vi "monitor_center.vi"() -> (1 "yc":dbl, 2 "xc":dbl)   [LabVIEW 2010]
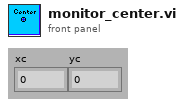
[diagram p1: front panel]
types:
  T1 = typedef "LVAllMonitorsDisplayTypeDef.ctl" = cluster{"Bounds":cluster{"Left":i16, "Top":i16, "Right":i16, "Bottom":i16}, "Depth":i16}[]
  T2 = cluster{"Bounds":cluster{"Left":i16, "Top":i16, "Right":i16, "Bottom":i16}, "Depth":i16}
  T3 = cluster{"Left":i16, "Top":i16, "Right":i16, "Bottom":i16}
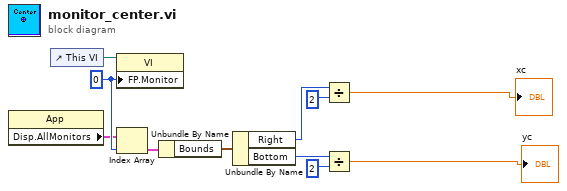
[diagram p0: block diagram]
diagram:
  w9 = u16 0 ("Front Panel Window:Monitor")
  n1 = property class="App"() -> ("Disp.AllMonitors"=w8:T1)  [unwired: 2 in, 2 out]
  n2 = control-ref of="This VI"() -> (w11:refnum<vi>)
  n3 = property class="VI"(reference=w11, "FP.Monitor"=w9) -> ()  [unwired: 1 in, 2 out]
  n4 = Index Array(array=w8, index=w9) -> (element=w10:T2)
  n5 = Unbundle By Name(w10) -> ("Bounds"=w7:T3)
  n6 = Unbundle By Name(w7) -> ("Right"=w6:i16, "Bottom"=w3:i16)
  n7 = Divide(x=w6, y=i16 2) -> (x/y=→"xc":dbl)
  n8 = Divide(x=w3, y=i16 2) -> (x/y=→"yc":dbl)
